vi "Init_queue.vi"(8 "error in (no error)":errorcluster, 9 "read queue":T1, 10 "Send queues":T2[](array[typedef]), 11 "QueueReader in":refnum<class "MultiQueueReader.lvclass">) -> (0 "error out":errorcluster, 3 "QueueReader out":refnum<class "MultiQueueReader.lvclass">)   [LabVIEW 2013, in "MultiQueueReader.lvclass"]
doc: "Initializes the reader. Call before first use"
uses:
  MultiQueueReader.lvclass
  message_queue.ctl
  Message/BaseMessage/BaseMessage.lvclass
  response queue.ctl
  response.ctl
  driver_status.ctl
  MultiQueueReader.lvclass/MultiQueueReader.ctl
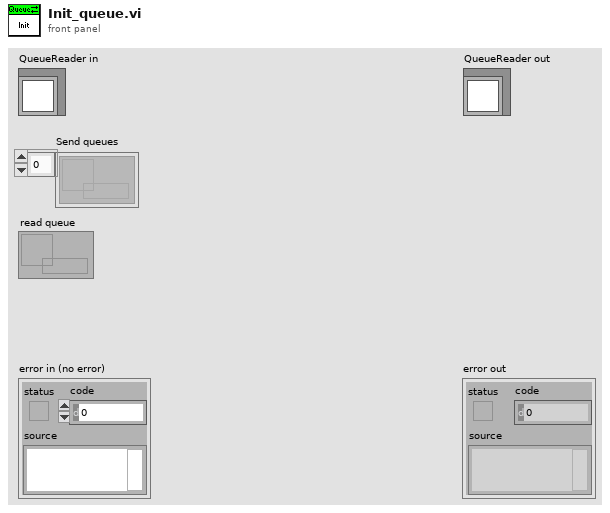
[diagram p1: front panel]
types:
  T1 = typedef "response queue.ctl" = refnum<queue>
  T2 = typedef "message_queue.ctl" = refnum<queue>
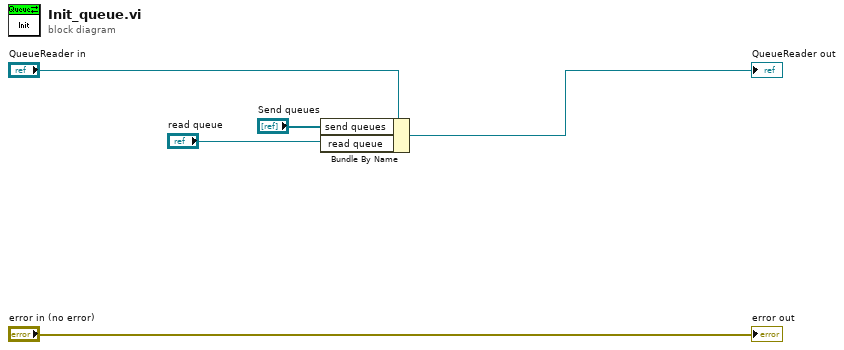
[diagram p0: block diagram]
diagram:
  n1 = Bundle By Name(cluster="QueueReader in", "send queues"="Send queues", "read queue"="read queue") -> (→"QueueReader out":refnum<class "MultiQueueReader.lvclass">)
  "error out" <- "error in (no error)"
